vi "CRYAPI MARK.vi"(0 "sAction":string="asada", 1 "mVritual_VIRef":refnum<vi>, 2 "sData":string="asada", 3 "MousePos":T1) -> (10 "bResult":bool=TRUE)   [LabVIEW 2013]
uses:
  <vilib>/Utility/miscctls.llb/LVRectTypeDef.ctl
  CRYMain Sub Window Global.vi
panel:
  in  "Rect_Main":T2
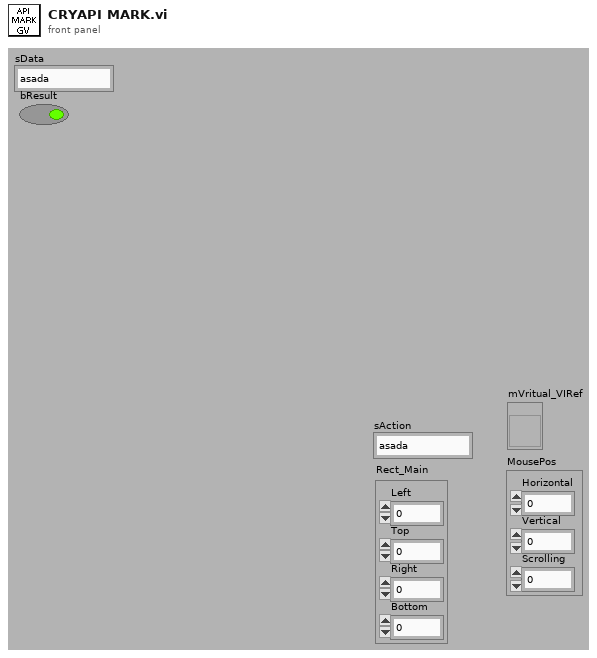
[diagram p1: front panel]
types:
  T1 = cluster{"Horizontal":i32, "Vertical":i32, "Scrolling":i32}
  T2 = typedef "LVRectTypeDef.ctl" = cluster{"Left":i16, "Top":i16, "Right":i16, "Bottom":i16}
  T3 = enum32{"Invalid", "Standard", "Closed", "Hidden", "Minimized", "Maximized"}
  T4 = enum32{"Invalid", "Default", "Floating", "Floating/Auto-Hide", "Modal"}
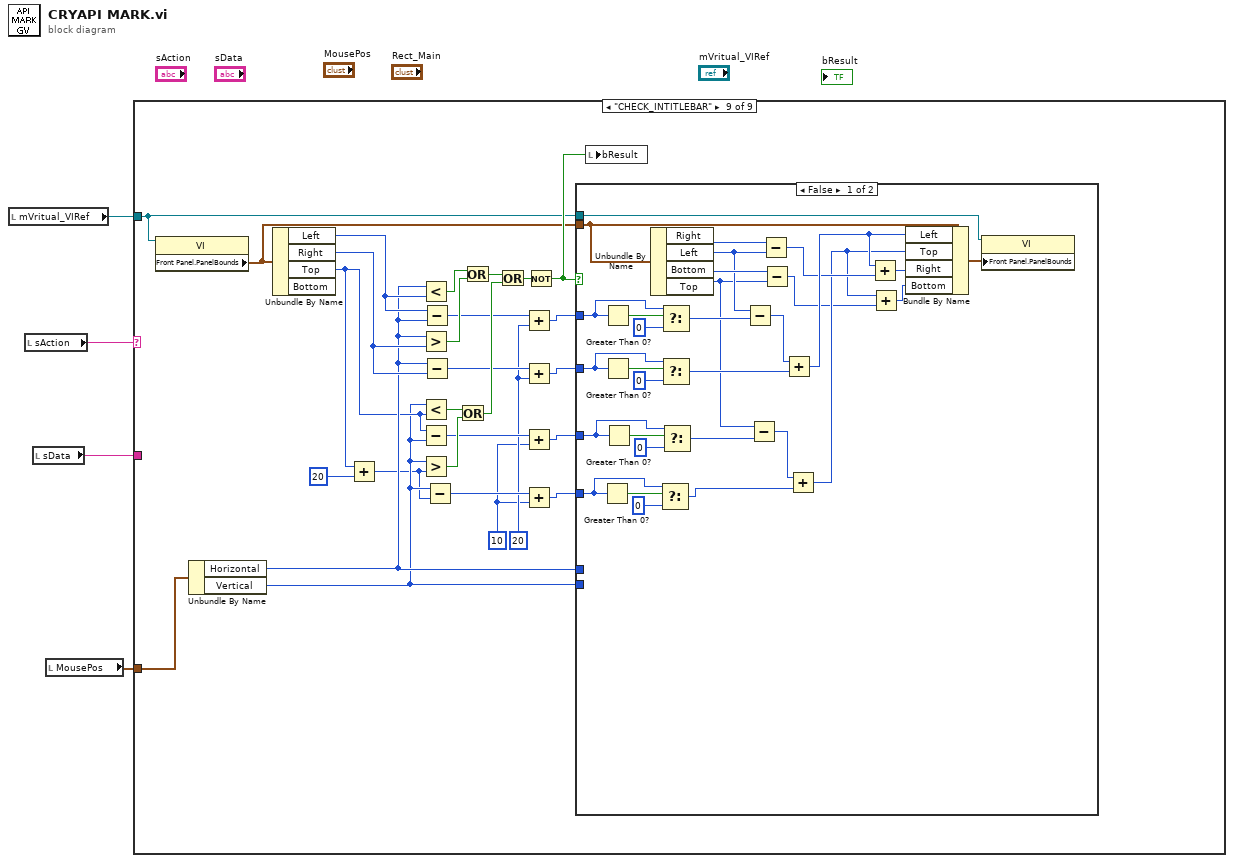
[diagram p0: block diagram]
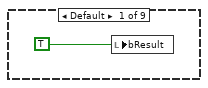
[diagram p2: hidden frame]
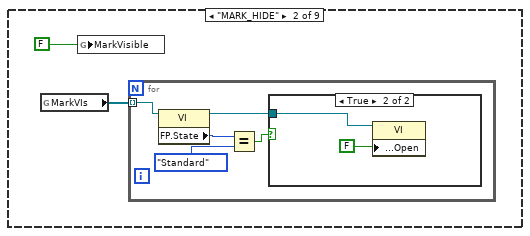
[diagram p3: hidden frame]
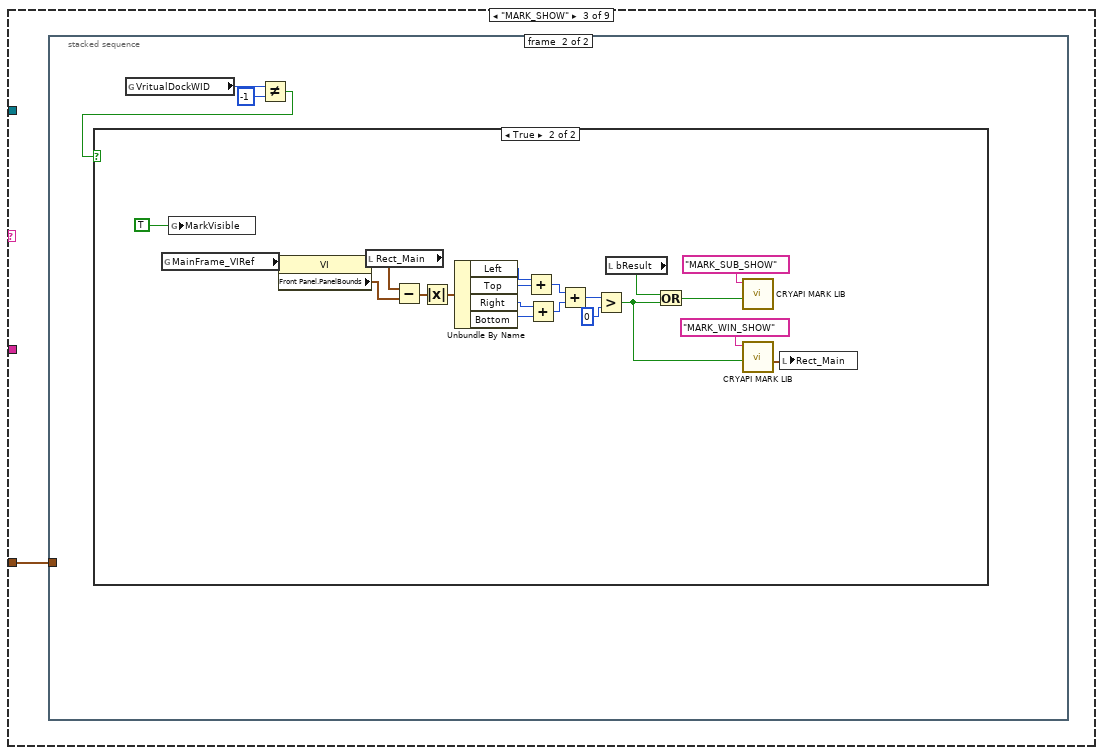
[diagram p5: hidden frame]
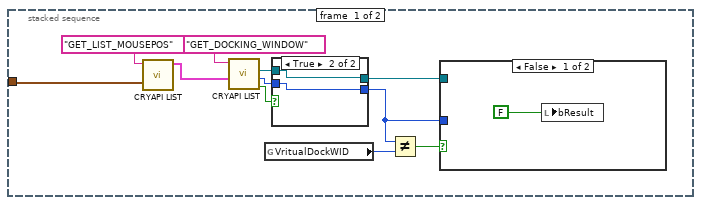
[diagram p6: hidden frame]
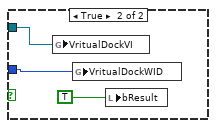
[diagram p7: hidden frame]
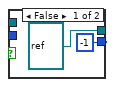
[diagram p8: hidden frame]
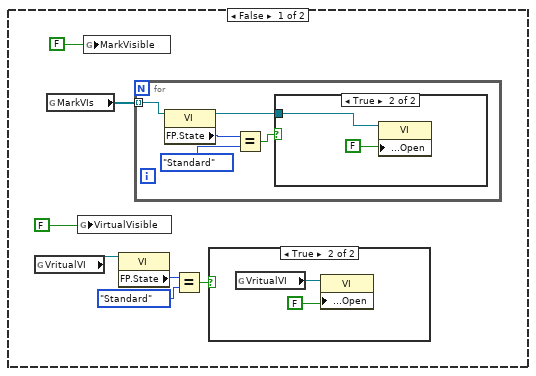
[diagram p9: hidden frame]
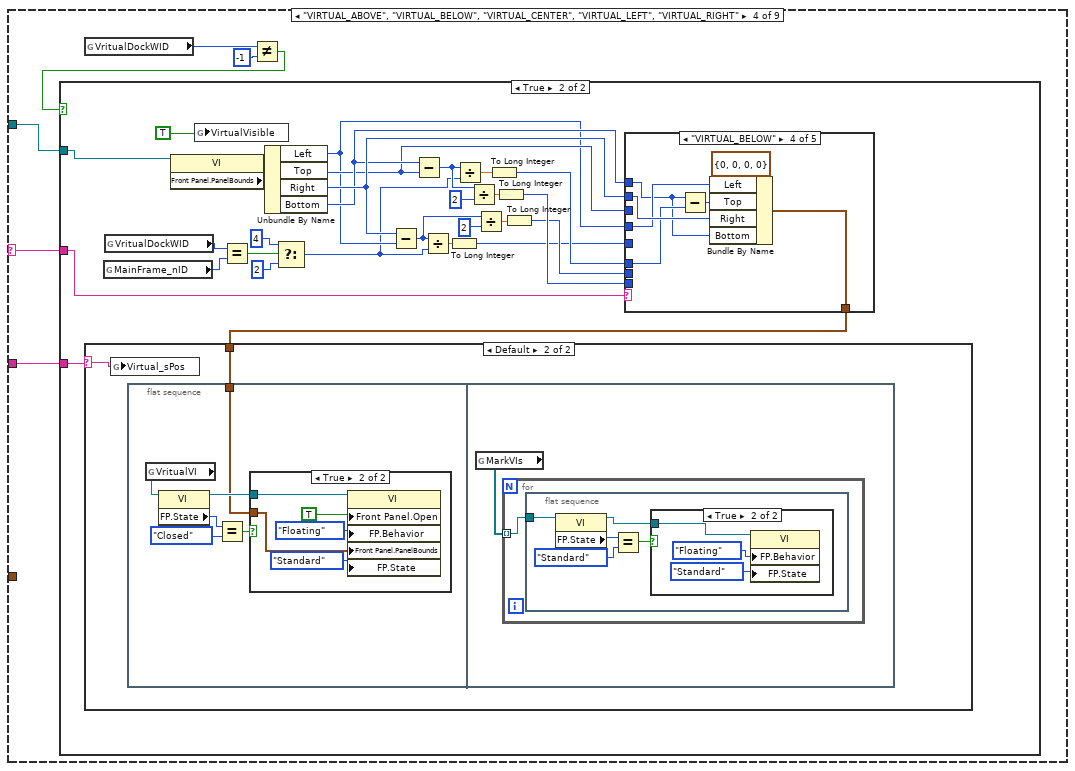
[diagram p12: hidden frame]
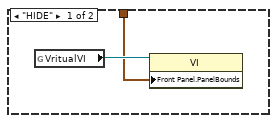
[diagram p14: hidden frame]
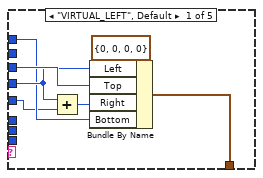
[diagram p17: hidden frame]
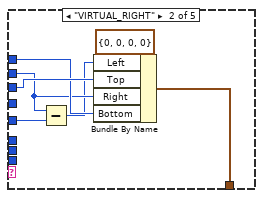
[diagram p18: hidden frame]
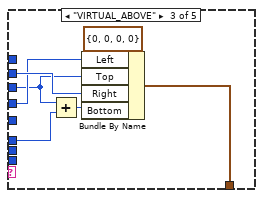
[diagram p19: hidden frame]
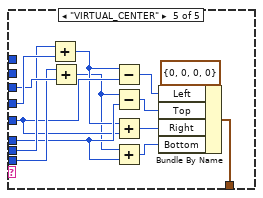
[diagram p20: hidden frame]
diagram:
  n1 = local read "mVritual_VIRef"() -> (w2:refnum<vi>)
  n2 = local read "sAction"() -> (w4:string)
  n3 = local read "sData"() -> (w1:string)
  n4 = local read "MousePos"() -> (w3:T1)
  n5 = case shown="\"CHECK_INTITLEBAR\"" w4 {
    selector: w4 -> [_ _ _ w79 _ _ _ _ _]
    tunnel: w3 -> [_ _ w15 _ _ w184 w218 w223 w268]
    tunnel: w2 -> [_ _ _ w75 _ _ _ w221 w251]
    tunnel: w1 -> [_ _ _ w74 _ _ _ _ _]
    frame Default {
      n6 = local write "bResult"(TRUE ("bResult")) -> ()
    }
    frame "MARK_HIDE" {
      n7 = global read "CRYMain Sub Window Global.vi" "MarkVIs"() -> (w7:refnum<vi>[])
      n8 = global write "CRYMain Sub Window Global.vi" "MarkVisible"(FALSE ("Mark VI State")) -> ()
      n9 = for {
        tunnel: w7 -> [w9] mode=indexing
        n10 = property class="VI"(reference=w9) -> (reference out=w8:refnum<vi>, "FP.State"=w12:T3)  [unwired: 1 in, 1 out]
        n11 = Equal?(x=w12, y=T3."Standard" ("Front Panel Window:State")) -> (x = y?=w10:bool)
        n12 = case shown="True" w10 {
          tunnel: w8 -> [_ w14]
          frame False {
          }
          frame True {
            n13 = property class="VI"(reference=w14, "Front Panel.Open"=FALSE ("Front Panel Window:Open")) -> ()  [unwired: 1 in, 2 out]
          }
        }
      }
    }
    frame "MARK_SHOW" {
      n14 = stacked-sequence {
        tunnel: w15 -> [w17 _]
        frame #0 {
          n15 = call "CRYAPI LIST.vi"("sAction"="GET_LIST_MOUSEPOS", "MousePos"=w17) -> ("List_Out"=w24:cluster{"nID":i32, "pVIRef":refnum<vi>}[])  [unwired: 2 in, 6 out]
          n16 = call "CRYAPI LIST.vi"("sAction"="GET_DOCKING_WINDOW", "List_In"=w24) -> ("pVIRef_Out"=w22:refnum<vi>, "nData_Out"=w18:i32, "bResult"=w23:bool)  [unwired: 2 in, 4 out]
          n17 = global read "CRYMain Sub Window Global.vi" "VritualDockWID"() -> (w21:i32)
          n18 = case shown="True" w23 {
            tunnel: w22 -> [_ w34]
            tunnel: [-1 w33] -> w19
            tunnel: [refnum<vi> refnum ("Vritual_Docking_VIRef") w34] -> w20
            tunnel: w18 -> [_ w33]
            frame False {
            }
            frame True {
            }
          }
          n19 = Not Equal?(x=w19, y=w21) -> (x != y?=w16:bool)
          n20 = case shown="False" w16 {
            tunnel: w20 -> [_ w30]
            tunnel: w19 -> [_ w29]
            frame False {
              n21 = local write "bResult"(FALSE ("Docking_Update")) -> ()
            }
            frame True {
              n22 = global write "CRYMain Sub Window Global.vi" "VritualDockVI"(w30) -> ()
              n23 = global write "CRYMain Sub Window Global.vi" "VritualDockWID"(w29) -> ()
              n24 = local write "bResult"(TRUE ("Docking_Update")) -> ()
            }
          }
        }
        frame #1 {
          n25 = global read "CRYMain Sub Window Global.vi" "VritualDockWID"() -> (w37:i32)
          n26 = Not Equal?(x=w37, y=-1) -> (x != y?=w35:bool)
          n27 = case shown="True" w35 {
            frame False {
              n28 = global read "CRYMain Sub Window Global.vi" "VritualVI"() -> (w39:refnum<vi>)
              n29 = global read "CRYMain Sub Window Global.vi" "MarkVIs"() -> (w43:refnum<vi>[])
              n30 = global write "CRYMain Sub Window Global.vi" "VirtualVisible"(FALSE ("VirtualVi")) -> ()
              n31 = global write "CRYMain Sub Window Global.vi" "MarkVisible"(FALSE ("Mark VI State")) -> ()
              n32 = property class="VI"(reference=w39) -> ("FP.State"=w41:T3)  [unwired: 1 in, 2 out]
              n33 = for {
                tunnel: w43 -> [w48] mode=indexing
                n34 = property class="VI"(reference=w48) -> (reference out=w47:refnum<vi>, "FP.State"=w51:T3)  [unwired: 1 in, 1 out]
                n35 = Equal?(x=w51, y=T3."Standard" ("Front Panel Window:State")) -> (x = y?=w49:bool)
                n36 = case shown="True" w49 {
                  tunnel: w47 -> [_ w53]
                  frame False {
                  }
                  frame True {
                    n37 = property class="VI"(reference=w53, "Front Panel.Open"=FALSE ("Front Panel Window:Open")) -> ()  [unwired: 1 in, 2 out]
                  }
                }
              }
              n38 = Equal?(x=w41, y=T3."Standard" ("Front Panel Window:State")) -> (x = y?=w40:bool)
              n39 = case shown="True" w40 {
                frame False {
                }
                frame True {
                  n40 = global read "CRYMain Sub Window Global.vi" "VritualVI"() -> (w46:refnum<vi>)
                  n41 = property class="VI"(reference=w46, "Front Panel.Open"=FALSE ("Front Panel Window:Open")) -> ()  [unwired: 1 in, 2 out]
                }
              }
            }
            frame True {
              n42 = global read "CRYMain Sub Window Global.vi" "MainFrame_VIRef"() -> (w61:refnum<vi>)
              n43 = global write "CRYMain Sub Window Global.vi" "MarkVisible"(TRUE ("Mark VI State")) -> ()
              n44 = property class="VI"(reference=w61) -> ("Front Panel.PanelBounds"=w60:T2)  [unwired: 1 in, 2 out]
              n45 = local read "Rect_Main"() -> (w73:T2)
              n46 = Subtract(x=w73, y=w60) -> (x-y=w66:T2)
              n47 = Absolute Value(x=w66) -> (abs(x)=w65:T2)
              n48 = Unbundle By Name(w65) -> ("Left"=w67:i16, "Top"=w70:i16, "Right"=w69:i16, "Bottom"=w68:i16)
              n49 = Add(x=w67, y=w70) -> (x+y=w71:i16)
              n50 = Add(x=w69, y=w68) -> (x+y=w72:i16)
              n51 = Add(x=w71, y=w72) -> (x+y=w64:i16)
              n52 = Greater?(x=w64, y=0) -> (0:w54:bool)
              n53 = local read "bResult"() -> (w57:bool)
              n54 = Or(x=w57, y=w54) -> (x .or. y?=w58:bool)
              n55 = call "CRYAPI MARK LIB.vi"("sAction"="MARK_SUB_SHOW", "Docking_Update"=w58) -> ()  [unwired: 1 in, 8 out]
              n56 = call "CRYAPI MARK LIB.vi"("sAction"="MARK_WIN_SHOW", "Docking_Update"=w54) -> ("Rect_Out"=w55:T2)  [unwired: 1 in, 7 out]
              n57 = local write "Rect_Main"(w55) -> ()
            }
          }
        }
      }
    }
    frame "VIRTUAL_ABOVE", "VIRTUAL_BELOW", "VIRTUAL_CENTER", "VIRTUAL_LEFT", "VIRTUAL_RIGHT" {
      n58 = global read "CRYMain Sub Window Global.vi" "VritualDockWID"() -> (w78:i32)
      n59 = Not Equal?(x=w78, y=-1) -> (x != y?=w76:bool)
      n60 = case shown="True" w76 {
        tunnel: w79 -> [_ w90]
        tunnel: w75 -> [_ w106]
        tunnel: w74 -> [_ w80]
        frame False {
        }
        frame True {
          n61 = global read "CRYMain Sub Window Global.vi" "MainFrame_nID"() -> (w95:i32)
          n62 = global read "CRYMain Sub Window Global.vi" "VritualDockWID"() -> (w89:i32)
          n63 = property class="VI"(reference=w106) -> ("Front Panel.PanelBounds"=w99:T2)  [unwired: 1 in, 2 out]
          n64 = global write "CRYMain Sub Window Global.vi" "VirtualVisible"(TRUE ("Virtual_State_Up")) -> ()
          n65 = Equal?(x=w89, y=w95) -> (x = y?=w94:bool)
          n66 = Unbundle By Name(w99) -> ("Left"=w97:i16, "Top"=w98:i16, "Right"=w105:i16, "Bottom"=w104:i16)
          n67 = Select(t=4, s=w94, f=2) -> (s? t:f=w91:i32)
          n68 = Subtract(x=w105, y=w97) -> (x-y=w100:i16)
          n69 = Subtract(x=w104, y=w98) -> (x-y=w103:i16)
          n70 = Divide(x=w100, y=w91) -> (x/y=w82:dbl)
          n71 = To Long Integer(number=w82) -> (32bit integer=w81:i32)
          n72 = Divide(x=w103, y=w91) -> (x/y=w88:dbl)
          n73 = Divide(x=w103, y=2) -> (x/y=w86:dbl)
          n74 = Divide(x=w100, y=2) -> (x/y=w84:dbl)
          n75 = To Long Integer(number=w88) -> (32bit integer=w87:i32)
          n76 = To Long Integer(number=w86) -> (32bit integer=w85:i32)
          n77 = To Long Integer(number=w84) -> (32bit integer=w83:i32)
          n78 = case shown="\"VIRTUAL_BELOW\"" w90 {
            tunnel: w97 -> [w137 _ w151 w158 w173]
            tunnel: w98 -> [w138 w145 w150 _ w172]
            tunnel: w105 -> [_ w143 w152 w159 _]
            tunnel: w104 -> [w135 w144 _ w156 _]
            tunnel: w81 -> [w134 w142 _ _ w164]
            tunnel: [w133 w140 w147 w154 w161] -> w107
            tunnel: w87 -> [_ _ w149 w157 w165]
            tunnel: w83 -> [_ _ _ _ w167]
            tunnel: w85 -> [_ _ _ _ w166]
            frame "VIRTUAL_LEFT", Default {
              n79 = Add(x=w137, y=w134) -> (x+y=w136:i32)
              n80 = Bundle By Name(cluster=T2 {"Left"=0, "Top"=0, "Right"=0, "Bottom"=0} ("Front Panel Window:Panel Bounds"), "Left"=w137, "Top"=w138, "Right"=w136, "Bottom"=w135) -> (w133:T2)
            }
            frame "VIRTUAL_RIGHT" {
              n81 = Subtract(x=w143, y=w142) -> (x-y=w141:i32)
              n82 = Bundle By Name(cluster=T2 {"Left"=0, "Top"=0, "Right"=0, "Bottom"=0} ("Front Panel Window:Panel Bounds"), "Left"=w141, "Top"=w145, "Right"=w143, "Bottom"=w144) -> (w140:T2)
            }
            frame "VIRTUAL_ABOVE" {
              n83 = Add(x=w150, y=w149) -> (x+y=w148:i32)
              n84 = Bundle By Name(cluster=T2 {"Left"=0, "Top"=0, "Right"=0, "Bottom"=0} ("Front Panel Window:Panel Bounds"), "Left"=w151, "Top"=w150, "Right"=w152, "Bottom"=w148) -> (w147:T2)
            }
            frame "VIRTUAL_BELOW" {
              n85 = Subtract(x=w156, y=w157) -> (x-y=w155:i32)
              n86 = Bundle By Name(cluster=T2 {"Left"=0, "Top"=0, "Right"=0, "Bottom"=0} ("Front Panel Window:Panel Bounds"), "Left"=w158, "Top"=w155, "Right"=w159, "Bottom"=w156) -> (w154:T2)
            }
            frame "VIRTUAL_CENTER" {
              n87 = Add(x=w167, y=w173) -> (x+y=w163:i32)
              n88 = Add(x=w166, y=w172) -> (x+y=w162:i32)
              n89 = Subtract(x=w163, y=w164) -> (x-y=w171:i32)
              n90 = Subtract(x=w162, y=w165) -> (x-y=w170:i32)
              n91 = Add(x=w163, y=w164) -> (x+y=w169:i32)
              n92 = Add(x=w162, y=w165) -> (x+y=w168:i32)
              n93 = Bundle By Name(cluster=T2 {"Left"=0, "Top"=0, "Right"=0, "Bottom"=0} ("Front Panel Window:Panel Bounds"), "Left"=w171, "Top"=w170, "Right"=w169, "Bottom"=w168) -> (w161:T2)
            }
          }
          n94 = case shown="Default" w80 {
            selector: w80 -> [_ w110]
            tunnel: w107 -> [w108 w111]
            frame "HIDE" {
              n95 = global read "CRYMain Sub Window Global.vi" "VritualVI"() -> (w109:refnum<vi>)
              n96 = property class="VI"(reference=w109, "Front Panel.PanelBounds"=w108) -> ()  [unwired: 1 in, 2 out]
            }
            frame Default {
              n97 = global write "CRYMain Sub Window Global.vi" "Virtual_sPos"(w110) -> ()
              n98 = flat-sequence {
                tunnel: w111 -> [w113]
                frame #0 {
                  n99 = global read "CRYMain Sub Window Global.vi" "VritualVI"() -> (w112:refnum<vi>)
                  n100 = property class="VI"(reference=w112) -> (reference out=w117:refnum<vi>, "FP.State"=w114:T3)  [unwired: 1 in, 1 out]
                  n101 = Equal?(x=w114, y=T3."Closed" ("Front Panel Window:State")) -> (x = y?=w116:bool)
                  n102 = case shown="True" w116 {
                    tunnel: w113 -> [_ w122]
                    tunnel: w117 -> [_ w119]
                    frame False {
                    }
                    frame True {
                      n103 = property class="VI"(reference=w119, "Front Panel.Open"=TRUE ("Front Panel Window:Open"), "FP.Behavior"=T4."Floating" ("Front Panel Window:Behavior"), "Front Panel.PanelBounds"=w122, "FP.State"=T3."Standard" ("Front Panel Window:State")) -> ()  [unwired: 1 in, 2 out]
                    }
                  }
                }
                frame #1 {
                  n104 = global read "CRYMain Sub Window Global.vi" "MarkVIs"() -> (w123:refnum<vi>[])
                  n105 = for {
                    tunnel: w123 -> [w124] mode=indexing
                    n106 = flat-sequence {
                      tunnel: w124 -> [w129]
                      frame #0 {
                        n107 = property class="VI"(reference=w129) -> (reference out=w125:refnum<vi>, "FP.State"=w128:T3)  [unwired: 1 in, 1 out]
                        n108 = Equal?(x=w128, y=T3."Standard" ("Front Panel Window:State")) -> (x = y?=w126:bool)
                        n109 = case shown="True" w126 {
                          tunnel: w125 -> [_ w130]
                          frame False {
                          }
                          frame True {
                            n110 = property class="VI"(reference=w130, "FP.Behavior"=T4."Floating" ("Front Panel Window:Behavior"), "FP.State"=T3."Standard" ("Front Panel Window:State")) -> ()  [unwired: 1 in, 2 out]
                          }
                        }
                      }
                    }
                  }
                }
              }
            }
          }
        }
      }
    }
    frame "VIRTUAL_HIDE" {
      n111 = global read "CRYMain Sub Window Global.vi" "VritualVI"() -> (w180:refnum<vi>)
      n112 = global write "CRYMain Sub Window Global.vi" "VirtualVisible"(FALSE ("VirtualVi")) -> ()
      n113 = property class="VI"(reference=w180) -> ("FP.State"=w178:T3)  [unwired: 1 in, 2 out]
      n114 = Equal?(x=w178, y=T3."Standard" ("Front Panel Window:State")) -> (x = y?=w179:bool)
      n115 = global write "CRYMain Sub Window Global.vi" "Virtual_sPos"("" ("Virtual_sPos")) -> ()
      n116 = case shown="True" w179 {
        frame False {
        }
        frame True {
          n117 = global read "CRYMain Sub Window Global.vi" "VritualVI"() -> (w182:refnum<vi>)
          n118 = property class="VI"(reference=w182, "Front Panel.Open"=FALSE ("Front Panel Window:Open")) -> ()  [unwired: 1 in, 2 out]
        }
      }
    }
    frame "CHECK_INMARK" {
      n119 = global read "CRYMain Sub Window Global.vi" "MarkVIs"() -> (w185:refnum<vi>[])
      n120 = for {
        tunnel: w185 -> [w202] mode=indexing
        tunnel: w184 -> [w200]
        tunnel: [w186] -> w183
        stop <- w186 stop-if-true
        n121 = Unbundle By Name(w200) -> ("Horizontal"=w199:i32, "Vertical"=w190:i32)
        n122 = property class="VI"(reference=w202) -> ("Front Panel.PanelBounds"=w201:T2)  [unwired: 1 in, 2 out]
        n123 = Unbundle By Name(w201) -> ("Left"=w198:i16, "Right"=w197:i16, "Top"=w196:i16, "Bottom"=w195:i16)
        n124 = Less?(x=w199, y=w198) -> (x < y?=w194:bool)
        n125 = Greater?(x=w199, y=w197) -> (0:w192:bool)
        n126 = Less?(x=w190, y=w196) -> (x < y?=w193:bool)
        n127 = Greater?(x=w190, y=w195) -> (0:w191:bool)
        n128 = Or(x=w194, y=w192) -> (x .or. y?=w188:bool)
        n129 = Or(x=w193, y=w191) -> (x .or. y?=w189:bool)
        n130 = Or(x=w188, y=w189) -> (x .or. y?=w187:bool)
        n131 = Not(x=w187) -> (.not. x?=w186:bool)
      }
      n132 = local write "bResult"(w183) -> ()
    }
    frame "CHECK_INMAIN" {
      n133 = global read "CRYMain Sub Window Global.vi" "MainFrame_VIRef"() -> (w219:refnum<vi>)
      n134 = Unbundle By Name(w218) -> ("Horizontal"=w215:i32, "Vertical"=w206:i32)
      n135 = property class="VI"(reference=w219) -> ("Front Panel.PanelBounds"=w216:T2)  [unwired: 1 in, 2 out]
      n136 = Unbundle By Name(w216) -> ("Left"=w214:i16, "Right"=w213:i16, "Top"=w212:i16, "Bottom"=w211:i16)
      n137 = Less?(x=w215, y=w214) -> (x < y?=w210:bool)
      n138 = Greater?(x=w215, y=w213) -> (0:w208:bool)
      n139 = Less?(x=w206, y=w212) -> (x < y?=w209:bool)
      n140 = Greater?(x=w206, y=w211) -> (0:w207:bool)
      n141 = Or(x=w210, y=w208) -> (x .or. y?=w204:bool)
      n142 = Or(x=w209, y=w207) -> (x .or. y?=w205:bool)
      n143 = Or(x=w204, y=w205) -> (x .or. y?=w203:bool)
      n144 = Not(x=w203) -> (.not. x?=w217:bool)
      n145 = local write "bResult"(w217) -> ()
    }
    frame "CHECK_INTABMENU" {
      n146 = Not Equal?(x=w221, y=refnum<vi> refnum) -> (x != y?=w222:bool)
      n147 = case shown="True" w222 {
        tunnel: w223 -> [_ w240]
        tunnel: w221 -> [_ w224]
        frame False {
        }
        frame True {
          n148 = Unbundle By Name(w240) -> ("Horizontal"=w237:i32, "Vertical"=w228:i32)
          n149 = property class="VI"(reference=w224) -> ("Front Panel.PanelBounds"=w238:T2)  [unwired: 1 in, 2 out]
          n150 = Unbundle By Name(w238) -> ("Left"=w236:i16, "Right"=w235:i16, "Top"=w234:i16, "Bottom"=w233:i16)
          n151 = Less?(x=w237, y=w236) -> (x < y?=w232:bool)
          n152 = Greater?(x=w237, y=w235) -> (0:w230:bool)
          n153 = Less?(x=w228, y=w234) -> (x < y?=w231:bool)
          n154 = Greater?(x=w228, y=w233) -> (0:w229:bool)
          n155 = Or(x=w232, y=w230) -> (x .or. y?=w226:bool)
          n156 = Or(x=w231, y=w229) -> (x .or. y?=w227:bool)
          n157 = Or(x=w226, y=w227) -> (x .or. y?=w225:bool)
          n158 = Not(x=w225) -> (.not. x?=w239:bool)
          n159 = local write "bResult"(w239) -> ()
        }
      }
    }
    frame "CHECK_INTITLEBAR" {
      w241 = 10
      w242 = 20
      n160 = property class="VI"(reference=w251) -> ("Front Panel.PanelBounds"=w259:T2)  [unwired: 1 in, 2 out]
      n161 = Unbundle By Name(w268) -> ("Horizontal"=w255:i32, "Vertical"=w253:i32)
      n162 = Unbundle By Name(w259) -> ("Left"=w256:i16, "Right"=w257:i16, "Top"=w254:i16)  [unwired: 1 out]
      n163 = Add(x=w254, y=i16 20) -> (x+y=w252:i16)
      n164 = Less?(x=w255, y=w256) -> (x < y?=w267:bool)
      n165 = Greater?(x=w255, y=w257) -> (0:w265:bool)
      n166 = Less?(x=w253, y=w254) -> (x < y?=w266:bool)
      n167 = Subtract(x=w254, y=w253) -> (x-y=w244:i32)
      n168 = Greater?(x=w253, y=w252) -> (0:w258:bool)
      n169 = Subtract(x=w256, y=w255) -> (x-y=w249:i32)
      n170 = Subtract(x=w255, y=w257) -> (x-y=w245:i32)
      n171 = Subtract(x=w253, y=w252) -> (x-y=w243:i32)
      n172 = Or(x=w266, y=w258) -> (x .or. y?=w264:bool)
      n173 = Or(x=w267, y=w265) -> (x .or. y?=w263:bool)
      n174 = Or(x=w263, y=w264) -> (x .or. y?=w262:bool)
      n175 = Add(x=w249, y=w242) -> (x+y=w250:i32)
      n176 = Add(x=w245, y=w242) -> (x+y=w248:i32)
      n177 = Add(x=w244, y=w241) -> (x+y=w247:i32)
      n178 = Add(x=w243, y=w241) -> (x+y=w246:i32)
      n179 = Not(x=w262) -> (.not. x?=w260:bool)
      n180 = case shown="False" w260 {
        tunnel: w259 -> [w299 _]
        tunnel: w251 -> [w298 _]
        tunnel: w253 -> [_ _]
        tunnel: w255 -> [_ _]
        tunnel: w250 -> [w295 _]
        tunnel: w248 -> [w288 _]
        tunnel: w247 -> [w289 _]
        tunnel: w246 -> [w285 _]
        frame False {
          n181 = Greater Than 0?(x=w285) -> (x > 0?=w286:bool)
          n182 = Greater Than 0?(x=w295) -> (x > 0?=w296:bool)
          n183 = Greater Than 0?(x=w288) -> (x > 0?=w292:bool)
          n184 = Greater Than 0?(x=w289) -> (x > 0?=w291:bool)
          n185 = Unbundle By Name(w299) -> ("Right"=w284:i16, "Left"=w282:i16, "Bottom"=w283:i16, "Top"=w275:i16)
          n186 = Select(t=w285, s=w286, f=0) -> (s? t:f=w273:i32)
          n187 = Select(t=w295, s=w296, f=0) -> (s? t:f=w281:i32)
          n188 = Select(t=w288, s=w292, f=0) -> (s? t:f=w279:i32)
          n189 = Select(t=w289, s=w291, f=0) -> (s? t:f=w274:i32)
          n190 = Subtract(x=w282, y=w281) -> (x-y=w280:i32)
          n191 = Subtract(x=w275, y=w274) -> (x-y=w276:i32)
          n192 = Subtract(x=w284, y=w282) -> (x-y=w277:i16)
          n193 = Subtract(x=w283, y=w275) -> (x-y=w270:i16)
          n194 = Add(x=w280, y=w279) -> (x+y=w278:i32)
          n195 = Add(x=w276, y=w273) -> (x+y=w271:i32)
          n196 = Add(x=w278, y=w277) -> (x+y=w272:i32)
          n197 = Add(x=w271, y=w270) -> (x+y=w269:i32)
          n198 = Bundle By Name(cluster=w299, "Left"=w278, "Top"=w271, "Right"=w272, "Bottom"=w269) -> (w297:T2)
          n199 = property class="VI"(reference=w298, "Front Panel.PanelBounds"=w297) -> ()  [unwired: 1 in, 2 out]
        }
        frame True {
        }
      }
      n200 = local write "bResult"(w260) -> ()
    }
  }
